vi "revToFreq.vi"(8 "error in (no error)":errorcluster, 10 "Motor Possition":dbl, 11 "Motor in":refnum<class "Motor.lvclass">) -> (0 "error out":errorcluster, 2 "Frequency":dbl, 3 "Motor out":refnum<class "Motor.lvclass">)   [LabVIEW 2019, in "Motor.lvclass"]
uses:
  Motor.lvclass
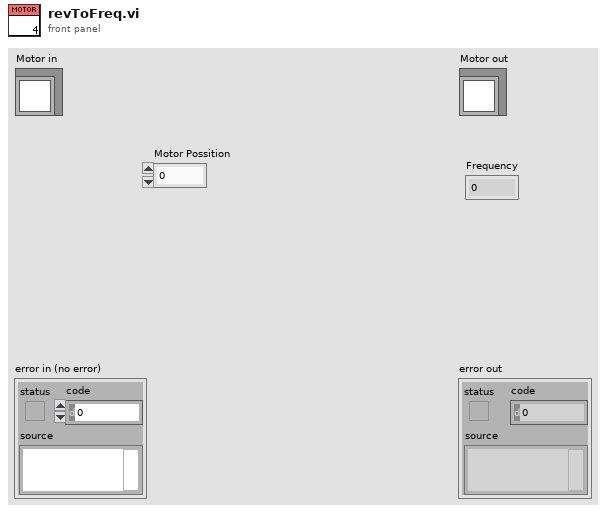
[diagram p1: front panel]
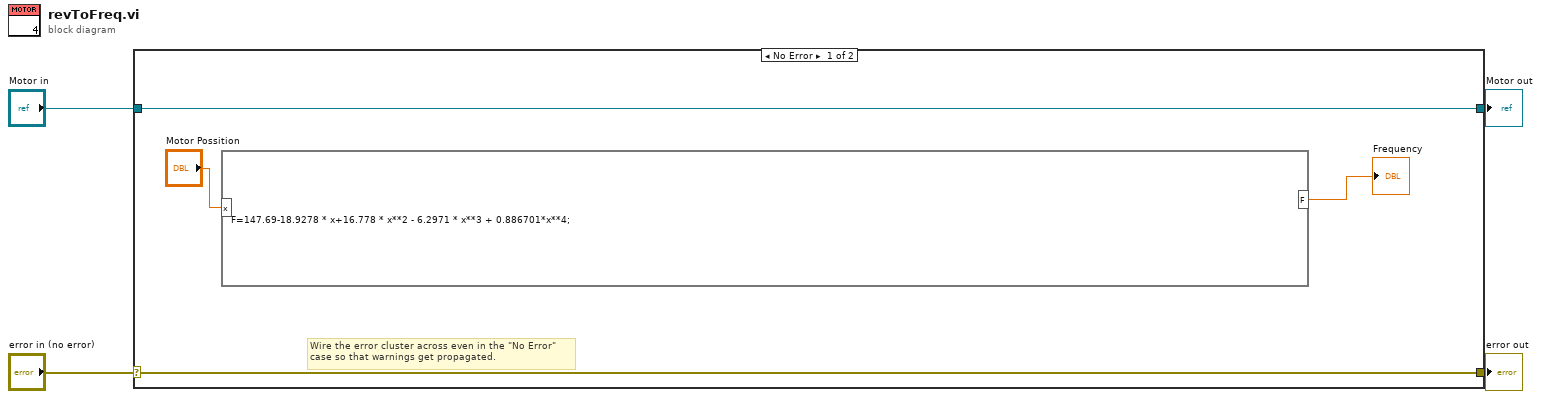
[diagram p0: block diagram]
diagram:
  n1 = case shown="No Error" "error in (no error)" {
    selector: "error in (no error)" -> [w7 w10]
    tunnel: [w7 w10] -> w3
    tunnel: [w8 w9] -> w1
    tunnel: "Motor in" -> [w8 w9]
    frame No Error {
      # "Wire the error cluster across even in the \"No Error\"\ncase so that warnings get propagated."
      n2 = formula code="F=147.69-18.9278 * x+16.778 * x**2 - 6.2971 * x**3 + 0.886701*x**4;"("x"="Motor Possition") -> ("F"=→"Frequency":dbl)
    }
    frame Error {
    }
  }
  "error out" <- w3
  "Motor out" <- w1
